vi "Case to Enum.vi"   [LabVIEW 2010]
panel:
  # "/* -------- Notes for All Users -------- */\nRecommand : \n[1].Display Setting Resolution -> 1440x900\n[2].Read Arch Notes First.\n[3].Make A Call When You Are In Trouble.\n\nTeam Members:\nGCC,GuFei,Jessie,LiuMing,TCC,ZSC\n\nCopyright@2010 Pansino.Beijing\n\nVersion Number: 3.0.0"
  # "/* -------- Notes for All Users -------- */\nRecommand : \n[1].Display Setting Resolution -> 1440x900\n[2].Read Arch Notes First.\n[3].Make A Call When You Are In Trouble.\n\nTeam Members:\nGCC,GuFei,Jessie,LiuMing,TCC,ZSC\n\nCopyright@2010 Pansino.Beijing\n\nVersion Number: 3.0.0"
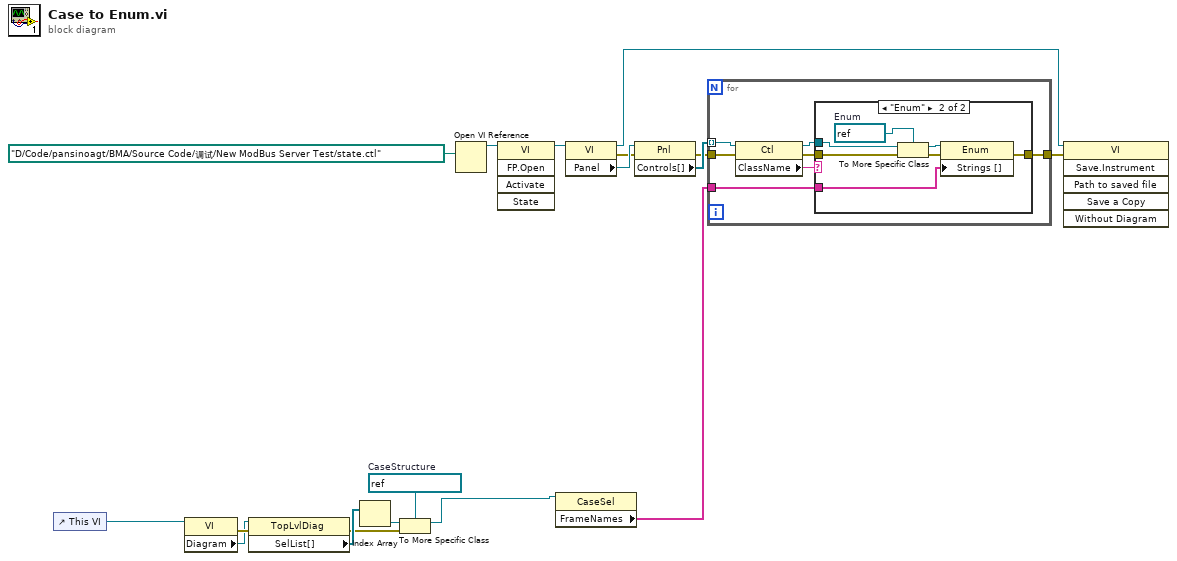
[diagram p0: block diagram]
diagram:
  w8 = refnum<vi> refnum  # CaseStructure
  n1 = control-ref of="This VI"() -> (w1:refnum<vi>)
  n2 = property class="VI"(reference=w1) -> (error out=w7:errorcluster, "Diagram"=w6:refnum<vi>)  [unwired: 1 in, 1 out]
  n3 = property class="TopLvlDiag"(reference=w6, error in=w7) -> (error out=w4:errorcluster, "SelList[]"=w5:refnum<vi>[])  [unwired: 1 out]
  n4 = Index Array(array=w5) -> (element=w9:refnum<vi>)  [unwired: 1 in]
  n5 = To More Specific Class(target class=w8, reference=w9, error in=w4) -> (specific class reference=w3:refnum<vi>)  [unwired: 1 out]
  n6 = Open VI Reference(vi path=path "D:/Code/pansinoagt/BMA/Source Code/调试/New ModBus Server Test/state.ctl") -> (vi reference=w15:refnum<vi>)  [unwired: 5 in, 1 out]
  n7 = invoke class="VI" method="FP.Open"(reference=w15) -> (reference out=w14:refnum<vi>)  [unwired: 4 in, 4 out]
  n8 = property class="CaseSel"(reference=w3) -> ("FrameNames"=w2:string[])  [unwired: 1 in, 2 out]
  n9 = property class="VI"(reference=w14) -> (reference out=w13:refnum<vi>, error out=w11:errorcluster, "Panel"=w17:refnum<vi>)  [unwired: 1 in]
  n10 = property class="Pnl"(reference=w17, error in=w11) -> (error out=w10:errorcluster, "Controls[]"=w16:refnum<vi>[])  [unwired: 1 out]
  n11 = for {
    tunnel: w16 -> [w25] mode=indexing
    tunnel: w2 -> [w22]
    tunnel: [w21] -> w12
    tunnel: w10 -> [w20]
    n12 = property class="Ctl"(reference=w25, error in=w20) -> (reference out=w23:refnum<vi>, error out=w19:errorcluster, "ClassName"=w24:string)
    n13 = case shown="\"Enum\"" w24 {
      tunnel: w23 -> [_ w33]
      tunnel: w22 -> [_ w30]
      tunnel: [w26 w29] -> w21
      tunnel: w19 -> [w26 w28]
      frame "False", Default {
      }
      frame "Enum" {
        w32 = refnum<vi> refnum  # Enum
        n14 = To More Specific Class(target class=w32, reference=w33, error in=w28) -> (specific class reference=w31:refnum<vi>, error out=w27:errorcluster)
        n15 = property class="Enum"(reference=w31, error in=w27, "Strings []"=w30) -> (error out=w29:errorcluster)  [unwired: 1 out]
      }
    }
  }
  n16 = invoke class="VI" method="Save.Instrument"(reference=w13, error in=w12) -> ()  [unwired: 4 in, 6 out]
